vi "testTimestampParsingZ.vi"(8 "error in (no error)":errorcluster, 11 "TestCase in":refnum<class "EasyXML_XML_Subset_Source_Tests.lvclass">) -> (0 "error out":errorcluster, 3 "TestCase out":refnum<class "EasyXML_XML_Subset_Source_Tests.lvclass">)   [LabVIEW 2013, in "EasyXML_XML_Subset_Source_Tests.lvclass"]
doc: "Verify that error in is not overwritten"
uses:
  EasyXML_XML_Subset_Source_Tests.lvclass
  EasyXML_XML_Subset_Evaluations/EasyXML_XML_Subset_Evaluations.lvclass
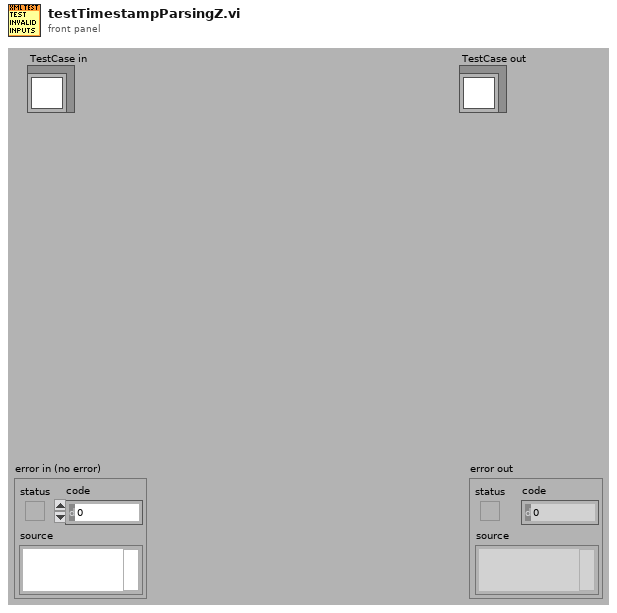
[diagram p1: front panel]
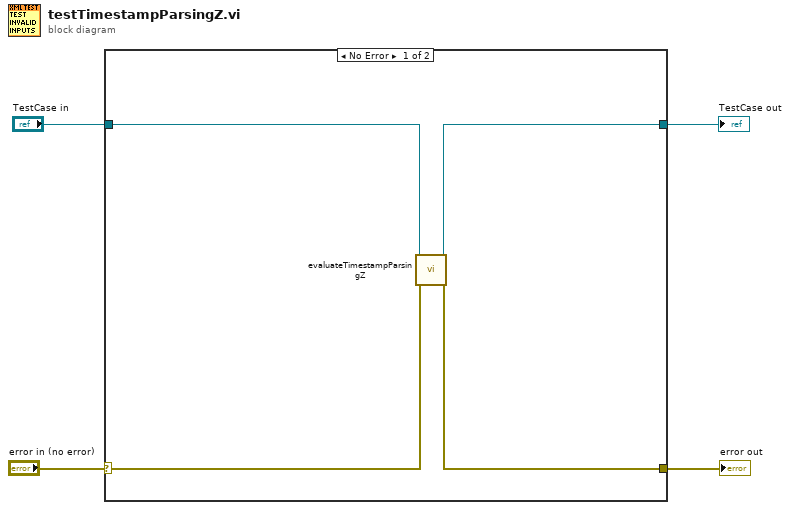
[diagram p0: block diagram]
diagram:
  n1 = case shown="No Error" "error in (no error)" {
    selector: "error in (no error)" -> [w7 w10]
    tunnel: [w6 w10] -> w2
    tunnel: [w5 w9] -> w1
    tunnel: "TestCase in" -> [w8 w9]
    frame No Error {
      n2 = call "evaluateTimestampParsingZ.vi"("error in (no error)"=w7, "TestCase in"=w8) -> ("error out"=w6:errorcluster, "TestCase out"=w5:refnum<class "EasyXML_XML_Subset_Source_Tests.lvclass">)  [unwired: 8 in]
    }
    frame Error {
    }
  }
  "error out" <- w2
  "TestCase out" <- w1
